vi "Non Linear Fit.vi"(10 "Integration Times":dbl[](array[numeric]), 11 "Slopes":dbl[](array[numeric])) -> (2 "Non Linear Model":dbl[](array[numeric]), 3 "Fit Verification":cluster{dbl[], "Best Power Fit":dbl[]}[](array[cluster]))   [LabVIEW 2014, in "AvaSpec.lvlib" / "Dark.lvlib"]
uses:
  Dark.lvlib
  <vilib>/gmath/NumericalOptimization/Nonlinear Curve Fit LM formula string.vi
  <vilib>/gmath/NI_Gmath.lvlib
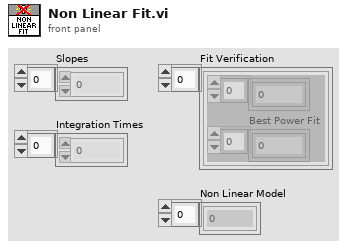
[diagram p1: front panel]
types:
  T1 = cluster{"model":string, "Parameters":string[], "x":string}
  T2 = cluster{"Integration Times":dbl[], "Slopes":dbl[]}
  T3 = cluster{"Integration Times":dbl[], "best nonlinear fit":dbl[]}
  T4 = cluster{"Integration Times":dbl[], "best nonlinear fit":dbl[]}[]
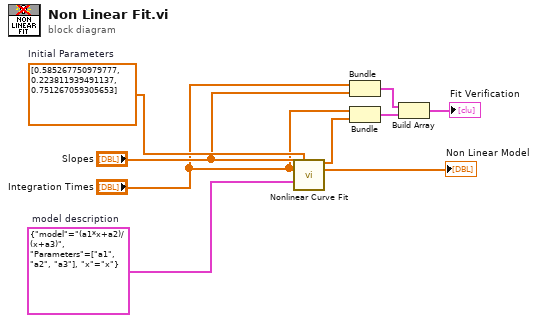
[diagram p0: block diagram]
diagram:
  w5 = dbl[] [0.585267750979777, 0.223811939491137, 0.751267059305653]  # Initial Parameters
  w6 = T1 {"model"="(a1*x+a2)/(x+a3)", "Parameters"=["a1", "a2", "a3"], "x"="x"}  # model description
  n1 = call-poly <vilib>:"Nonlinear Curve Fit.vi"("Y"="Slopes", "initial parameters"=w5, "X"="Integration Times", "model description"=w6) -> ("best nonlinear fit"=w4:dbl[], "best fit parameters"=→"Non Linear Model":dbl[])  [unwired: 7 in, 3 out]
  n2 = Bundle("Integration Times"="Integration Times", "Slopes"="Slopes") -> (w7:T2)  [unwired: 1 in]
  n3 = Bundle("Integration Times"="Integration Times", "best nonlinear fit"=w4) -> (w8:T3)  [unwired: 1 in]
  n4 = Build Array(w7, w8) -> (→"Fit Verification":T4)
